vi "PDE_State_Machine_12_12_ver_3.vi"() -> ()   [LabVIEW 2016]
uses:
  PDEState.ctl
  <vilib>/DAQmx/write.llb/DAQmx Write (Digital 1D Bool NChan 1Samp 1Line).vi
  <vilib>/DAQmx/read.llb/DAQmx Read (Analog 1D Wfm NChan NSamp).vi
  StateIndicator.ctl
  SubVIs/FireSlider.ctl
panel:
  out "error out":errorcluster
  out "Temperature":waveform(dbl)[](graph)
  out "PDE Progress":dbl(slide) scale=0.0..1.0
  out "Predet Progress":dbl(slide) scale=0.0..1.0
  in  "Number of Predet Fires":T1=1 min=0 max=100 step=1 scale=1.0..100.0
  out "Predet Fire Counter":i32
  out "Pressure":waveform(dbl)[](graph)
  out "PD Values":dbl[](array[numeric])
  out "PDE State":T2 items=["Stop VI", "Predet Fire", "Control Button", "Stop", "Connecting", "Firing", "Testing ", "Idle", "Init"]
  in  "Number of Fires":T1=1 min=0 max=100 step=1 scale=1.0..100.0
  out "Fire Counter":i32
  in  "Save Data":bool
  in  "Purge":bool=TRUE
  in  "Data Time":dbl=1.0 min=0.0 max=120.0
  in  "PT Filepath":path=path "D:/PDE Project/PDE Data/Default Data/PT.tdms"
  in  "TC Filepath":path=path "D:/PDE Project/PDE Data/Default Data/TC.tdms"
  in  "PD Filepath":path=path "D:/PDE Project/PDE Data/Default Data/PD.tdms"
  in  "Valve Buttons":bool[](array[boolean])
  in  "Predet Fire Button":bool
  in  "Control Buttons":bool
  in  "PDE Fire Button":bool
  in  "Test Button":bool
  in  "Go To Idle":bool
  in  "Abort VI":bool
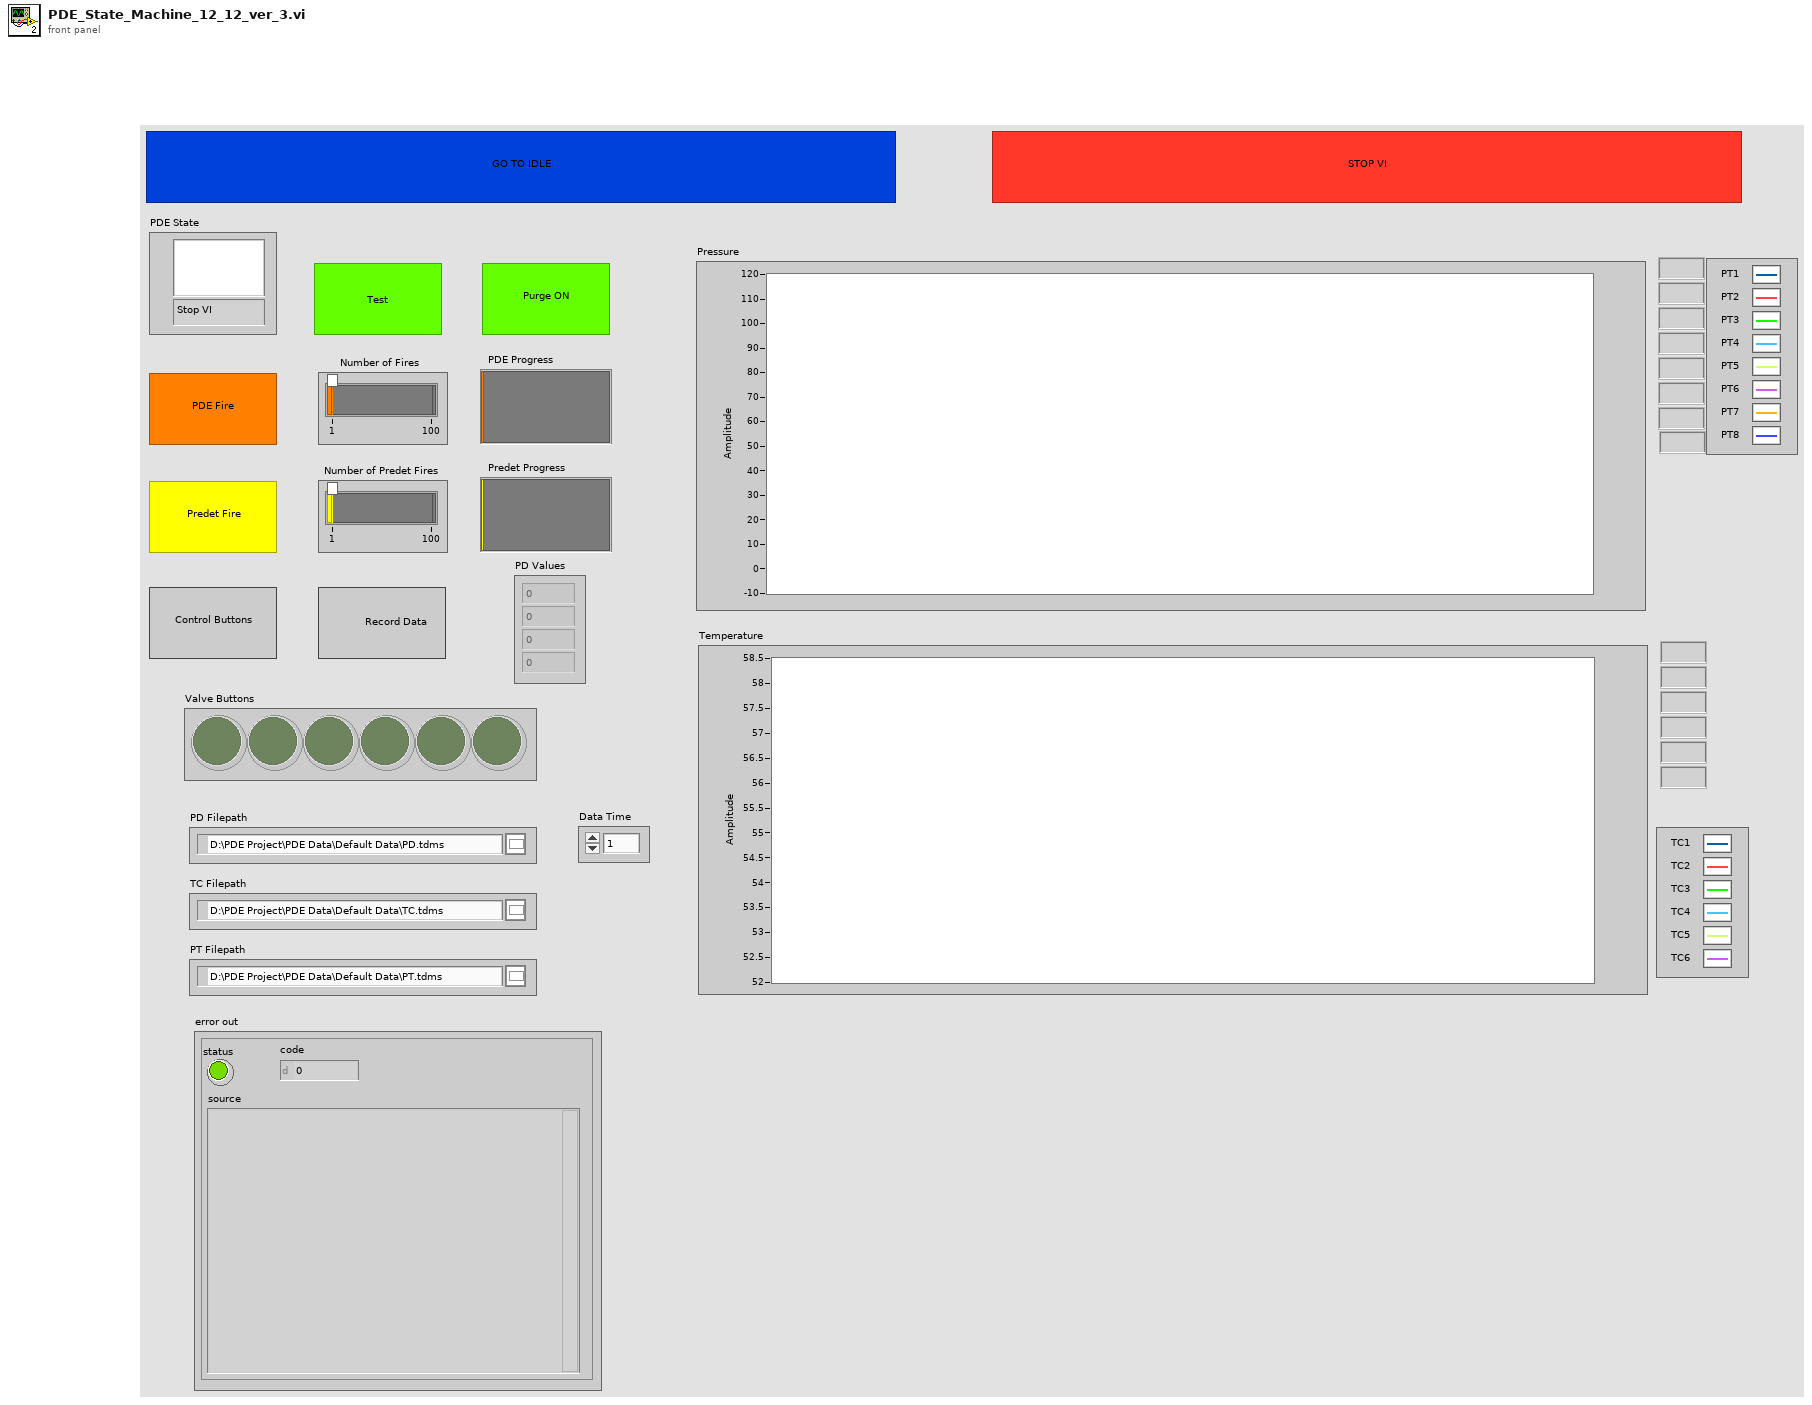
[diagram p1: front panel]
types:
  T1 = typedef "FireSlider.ctl" = i32
  T2 = typedef "StateIndicator.ctl" = u16
  T3 = typedef "PDEState.ctl" = enum16{"Stop VI", "Predet Fire", "Control Button", "Stop", "Connecting", "Firing ", "Testing ", "Idle", "Init"}
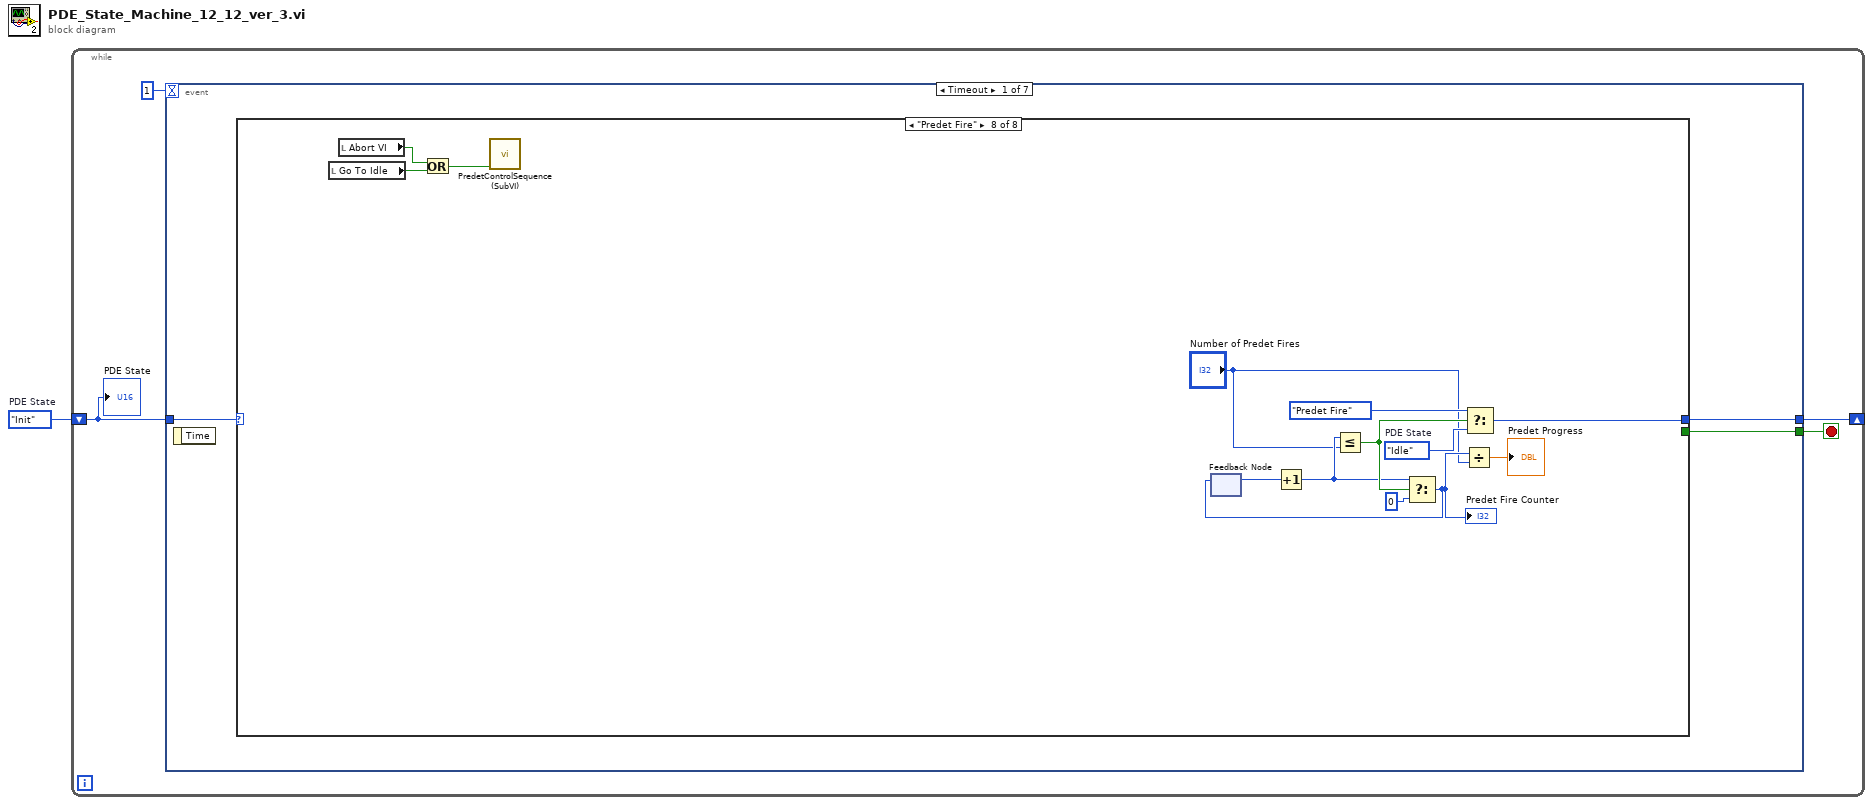
[diagram p0: block diagram]
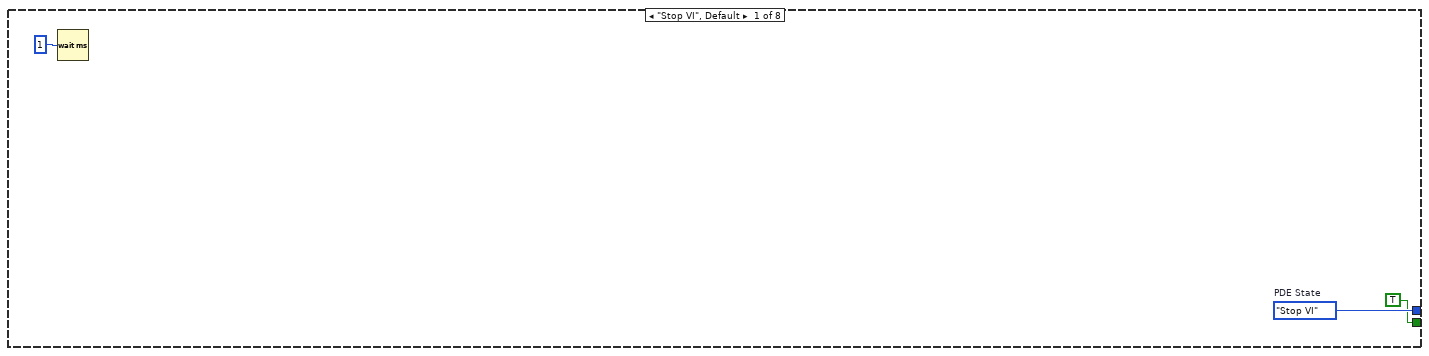
[diagram p2: hidden frame]
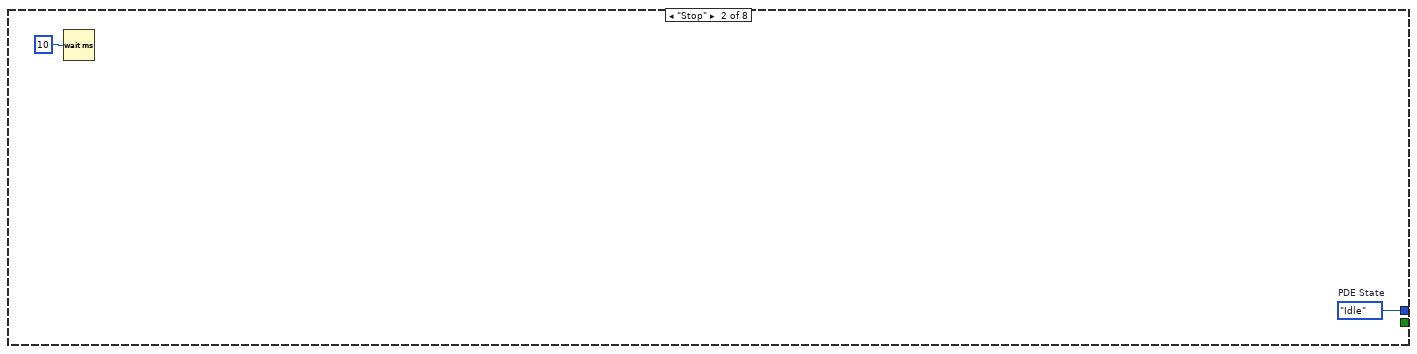
[diagram p3: hidden frame]
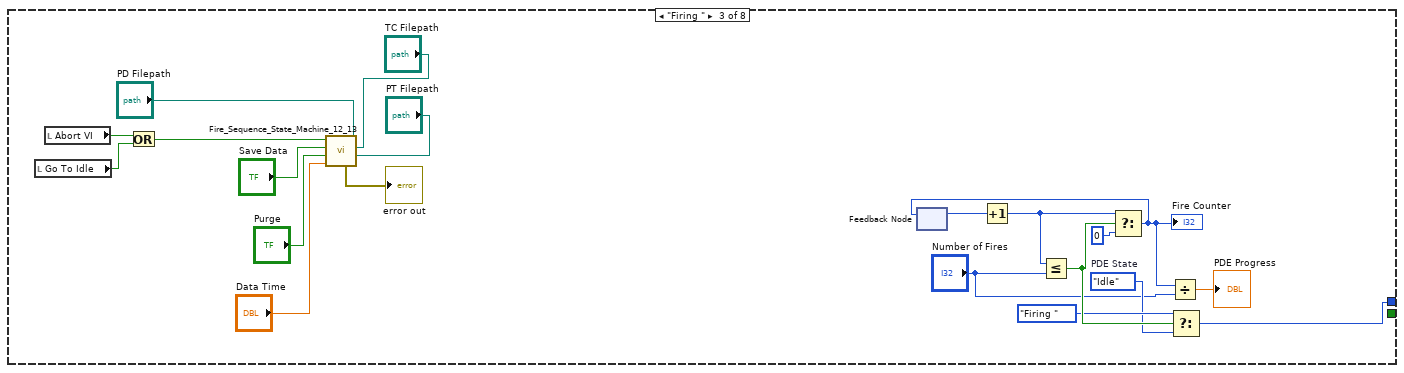
[diagram p4: hidden frame]
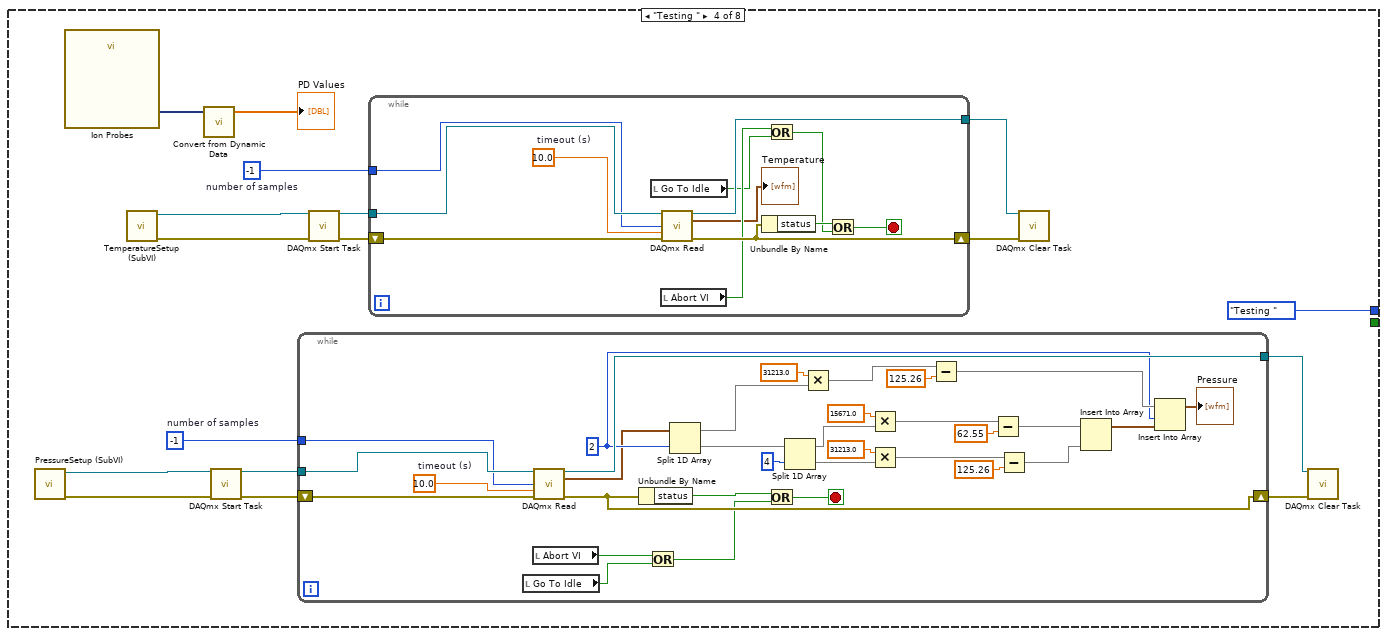
[diagram p5: hidden frame]
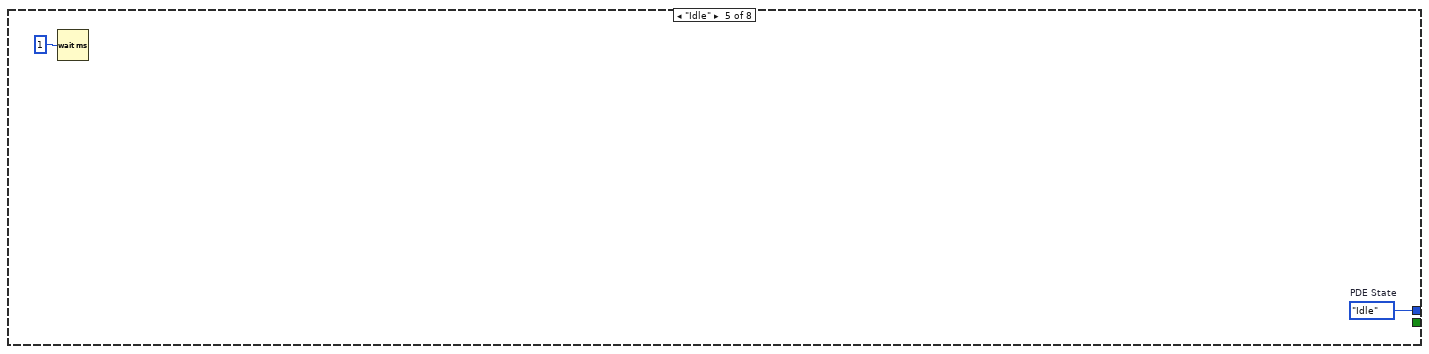
[diagram p6: hidden frame]
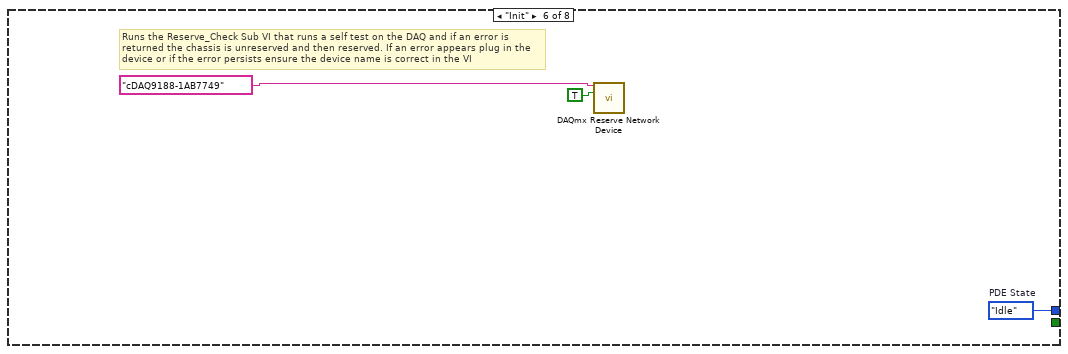
[diagram p7: hidden frame]
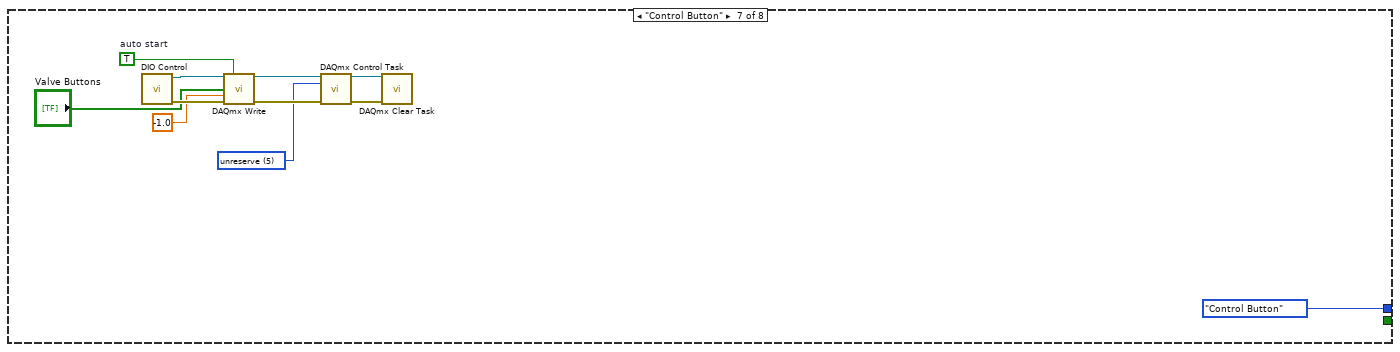
[diagram p8: hidden frame]
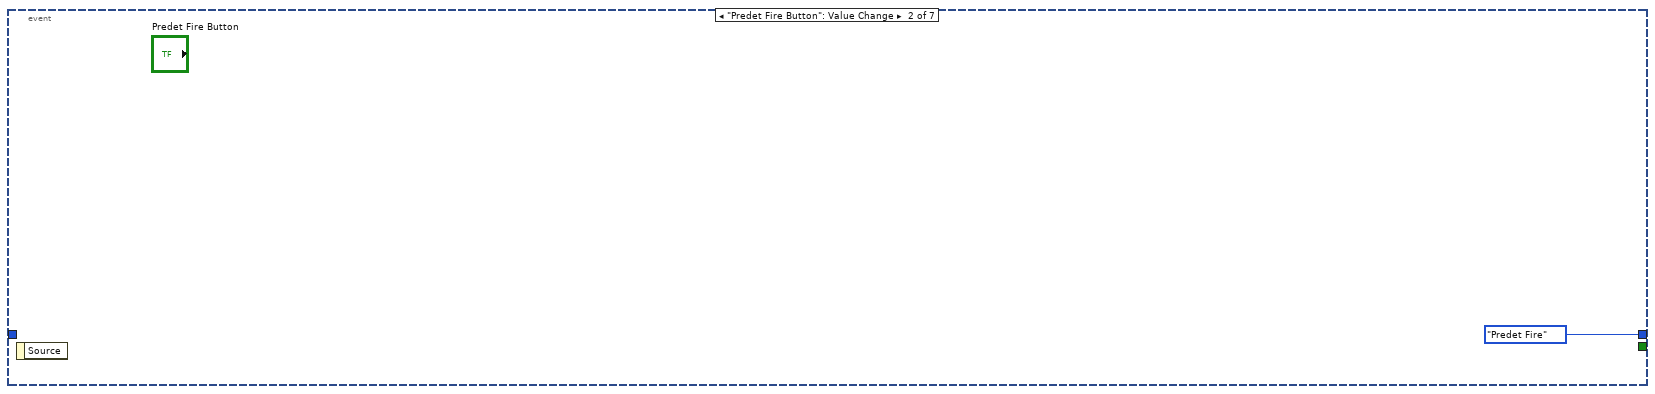
[diagram p9: hidden frame]
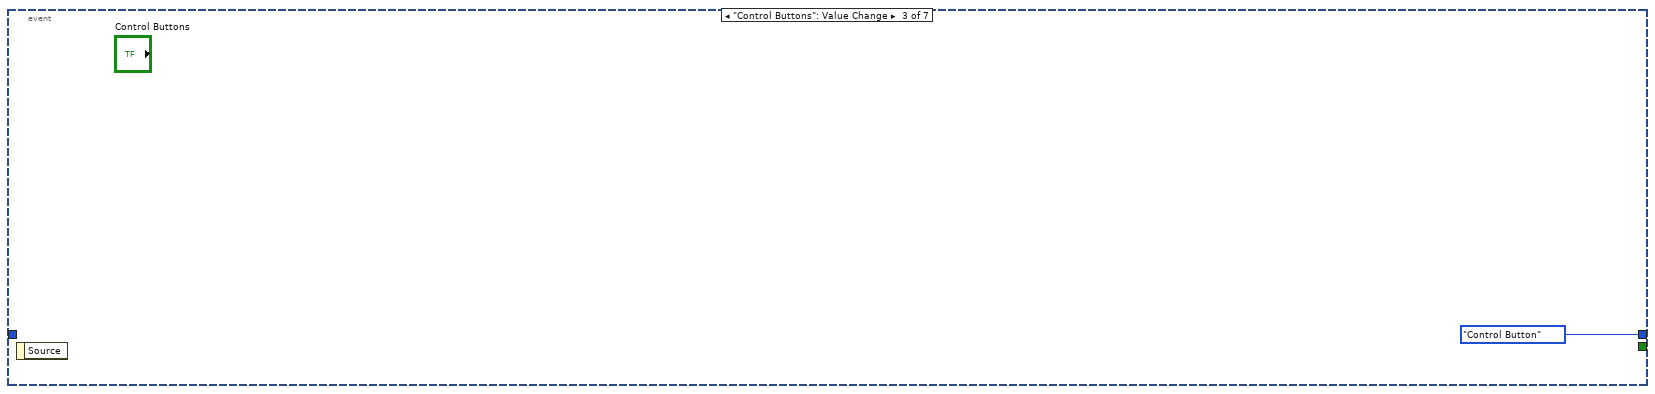
[diagram p10: hidden frame]
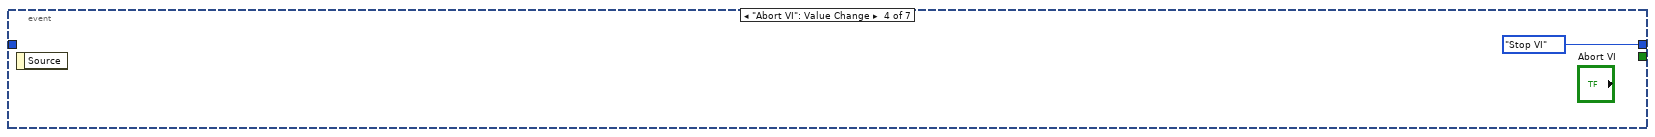
[diagram p11: hidden frame]
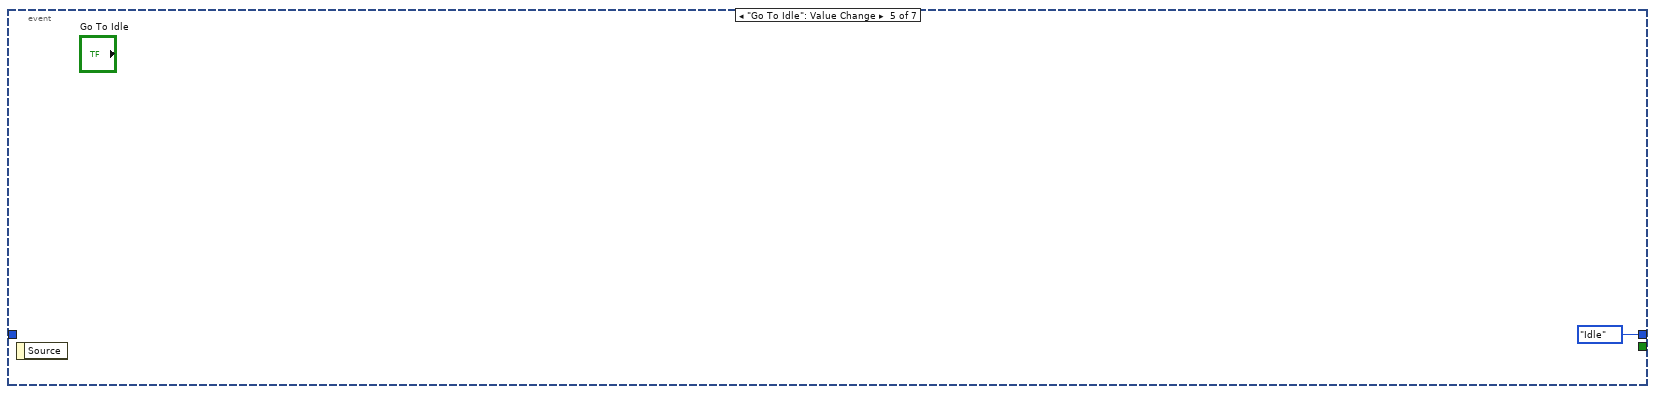
[diagram p12: hidden frame]
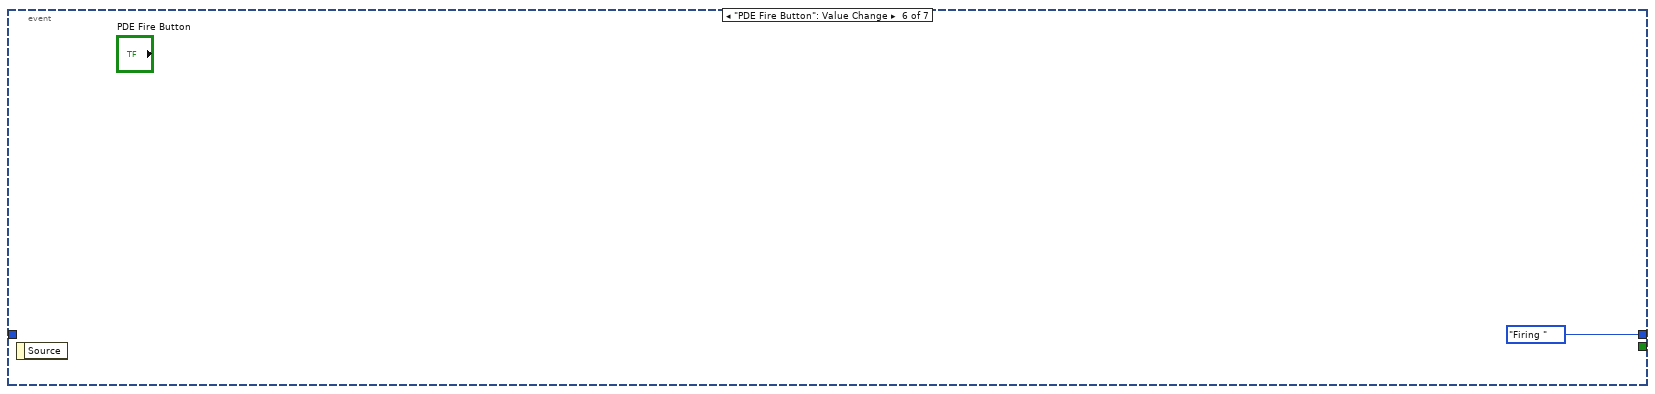
[diagram p13: hidden frame]
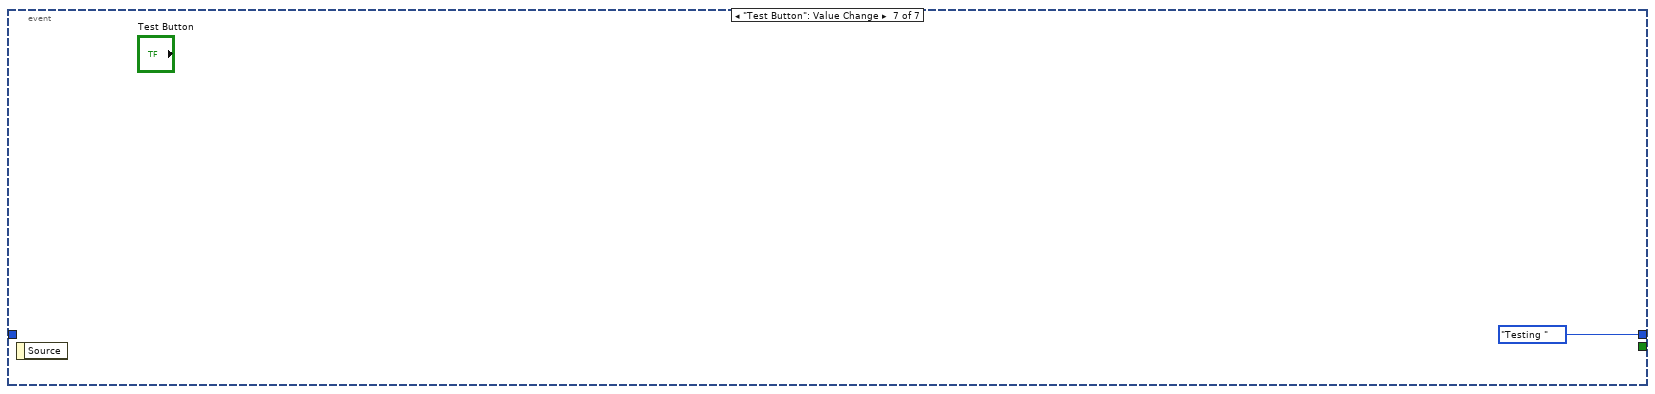
[diagram p14: hidden frame]
diagram:
  w1 = PDEState."Init"  # PDE State
  n1 = while {
    shift-right: [w4] -> _
    shift-left: w1 -> [w2]
    stop <- w3 stop-if-true
    n2 = event shown="[0] Timeout" {
      selector: _ -> [_ _ _ _ _ _ _]
      dyn-events: _ -> [_ _ _ _ _ _ _]
      timeout: 1 -> [_ _ _ _ _ _ _]
      tunnel: w2 -> [w8 _ _ _ _ _ _]
      tunnel: [w7 PDEState."Predet Fire" ("PDE State") PDEState."Control Button" ("PDE State") PDEState."Stop VI" ("PDE State") PDEState."Idle" ("PDE State") PDEState."Firing " ("PDE State") PDEState."Testing " ("PDE State")] -> w4
      tunnel: [w6 _ _ _ _ _ _] -> w3
      event Timeout {
        n3 = event-data() -> ()  [unwired: 1 in, 1 out]
        n4 = case shown="\"Predet Fire\"" w8 {
          tunnel: [w11 w13 w27 PDEState."Testing " ("PDE State") w96 w99 PDEState."Control Button" ("PDE State") w117] -> w7
          tunnel: [TRUE _ _ _ _ _ _ _] -> w6
          frame "Stop VI", Default {
            w11 = PDEState."Stop VI"  # PDE State
            n5 = Wait (ms)(milliseconds to wait=u32 1 ("millisecond timer value")) -> ()  [unwired: 1 out]
          }
          frame "Stop" {
            w13 = PDEState."Idle"  # PDE State
            n6 = Wait (ms)(milliseconds to wait=u32 10 ("millisecond timer value")) -> ()  [unwired: 1 out]
          }
          frame "Firing " {
            w28 = PDEState."Idle"  # PDE State
            n7 = local read "Go To Idle"() -> (w20:bool)
            n8 = local read "Abort VI"() -> (w19:bool)
            n9 = Or(x=w19, y=w20) -> (x .or. y?=w18:bool)
            n10 = call "Fire_Sequence_State_Machine_12_13.vi"("PT Filepath"="PT Filepath", "TC Filepath"="TC Filepath", "PD Filepath"="PD Filepath", "Data Time"="Data Time", "Purge"="Purge", "Save Data"="Save Data", "Stop Button"=w18) -> ("Error Out"=→"error out":errorcluster)  [unwired: 3 in, 1 out]
            n11 = feedback #1() -> (w31:i32)  [unwired: 1 in]
            n12 = Increment(x=w31) -> (x+1=w30:i32)
            n13 = Less Or Equal?(x=w30, y="Number of Fires") -> (x <= y?=w33:bool)
            n14 = Select(t=w30, s=w33, f=0 ("s? t:f")) -> (s? t:f=w16:i32)
            "Fire Counter" <- w16
            n15 = feedback-in #1(w16) -> ()
            n16 = Divide(x=w16, y="Number of Fires") -> (x/y=→"PDE Progress":dbl)
            n17 = Select(t=PDEState."Firing ", s=w33, f=w28) -> (s? t:f=w27:T3)
          }
          frame "Testing " {
            w38 = -1  # number of samples
            w46 = -1  # number of samples
            n18 = call "PressureSetup (SubVI).vi"() -> ("error out"=w42:errorcluster, "Refnum out"=w43:refnum<k21>)  [unwired: 10 in]
            n19 = call "Ion Probes"() -> ("data"=w49:dynamicdata)  [unwired: 17 in, 2 out]
            n20 = call "TemperatureSetup (SubVI).vi"() -> ("error out"=w34:errorcluster, "Refnum out"=w35:refnum<k21>)  [unwired: 10 in]
            n21 = call "Convert from Dynamic Data"("Dynamic Data Type"=w49) -> ("Array"=→"PD Values":dbl[])  [unwired: 3 in]
            n22 = call <vilib>:"DAQmx Start Task.vi"("task/channels in"=w43, "error in"=w42) -> ("task out"=w48:refnum<k21>, "error out"=w47:errorcluster)  [unwired: 12 out]
            n23 = while {
              tunnel: w48 -> [w94]
              tunnel: w46 -> [w91]
              tunnel: [w92] -> w44
              shift-right: [w89] -> w45
              shift-left: w47 -> [w93]
              stop <- w87 stop-if-true
              w75 = 2 ("index")
              w88 = 10.0  # timeout (s)
              n24 = local read "Go To Idle"() -> (w86:bool)
              n25 = local read "Abort VI"() -> (w85:bool)
              n26 = call-poly <vilib>:"DAQmx Read.vi"("task/channels in"=w94, "number of samples per channel"=w91, "timeout"=w88, "error in"=w93) -> ("task out"=w92:refnum<k21>, "data"=w74:waveform(dbl)[], "error out"=w89:errorcluster)  [unwired: 9 out]
              n27 = Unbundle By Name(w89) -> ("status"=w90:bool)
              n28 = Or(x=w85, y=w86) -> (x .or. y?=w84:bool)
              n29 = Split 1D Array(array=w74, index=w75) -> (first subarray=w80:waveform(dbl)[], second subarray=w72:waveform(dbl)[])
              n30 = Or(x=w90, y=w84) -> (x .or. y?=w87:bool)
              n31 = Split 1D Array(array=w72, index=4) -> (first subarray=w64:waveform(dbl)[], second subarray=w65:waveform(dbl)[])
              n32 = Multiply(x=31213.0, y=w80) -> (x*y=w83:waveform(dbl)[])
              n33 = Multiply(x=15671.0, y=w64) -> (x*y=w79:waveform(dbl)[])
              n34 = Multiply(x=31213.0, y=w65) -> (x*y=w70:waveform(dbl)[])
              n35 = Subtract(x=w83, y=125.26) -> (x-y=w76:waveform(dbl)[])
              n36 = Subtract(x=w79, y=62.55) -> (x-y=w63:waveform(dbl)[])
              n37 = Subtract(x=w70, y=125.26) -> (x-y=w66:waveform(dbl)[])
              n38 = Insert Into Array(array=w63, new element=w66) -> (w67:waveform(dbl)[])  [unwired: 1 in]
              n39 = Insert Into Array(array=w76, index=w75, new element=w67) -> (→"Pressure":waveform(dbl)[])
            }
            n40 = call <vilib>:"DAQmx Start Task.vi"("task/channels in"=w35, "error in"=w34) -> ("task out"=w40:refnum<k21>, "error out"=w39:errorcluster)  [unwired: 12 out]
            n41 = while {
              tunnel: w40 -> [w62]
              tunnel: w38 -> [w59]
              tunnel: [w60] -> w36
              shift-right: [w57] -> w37
              shift-left: w39 -> [w61]
              stop <- w56 stop-if-true
              w55 = 10.0  # timeout (s)
              n42 = local read "Go To Idle"() -> (w53:bool)
              n43 = local read "Abort VI"() -> (w54:bool)
              n44 = call-poly <vilib>:"DAQmx Read.vi"("task/channels in"=w62, "number of samples per channel"=w59, "timeout"=w55, "error in"=w61) -> ("task out"=w60:refnum<k21>, "data"=→"Temperature":waveform(dbl)[], "error out"=w57:errorcluster)  [unwired: 9 out]
              n45 = Unbundle By Name(w57) -> ("status"=w58:bool)
              n46 = Or(x=w54, y=w53) -> (x .or. y?=w52:bool)
              n47 = Or(x=w58, y=w52) -> (x .or. y?=w56:bool)
            }
            n48 = call <vilib>:"DAQmx Clear Task.vi"("task in"=w36, "error in"=w37) -> ()  [unwired: 14 out]
            n49 = call <vilib>:"DAQmx Clear Task.vi"("task in"=w44, "error in"=w45) -> ()  [unwired: 14 out]
          }
          frame "Idle" {
            w96 = PDEState."Idle"  # PDE State
            n50 = Wait (ms)(milliseconds to wait=u32 1 ("millisecond timer value")) -> ()  [unwired: 1 out]
          }
          frame "Init" {
            w99 = PDEState."Idle"  # PDE State
            # "Runs the Reserve_Check Sub VI that runs a self test on the DAQ and if an error is returned the chassis is unreserved and then reserved. If an error appears plug in the device or if the error persists ensure the device name is correct in the VI"
            n51 = call <vilib>:"DAQmx Reserve Network Device.vi"("device in"=tag "cDAQ9188-1AB7749", "override reservation?"=TRUE) -> ()  [unwired: 12 in, 2 out]
          }
          frame "Control Button" {
            w104 = 5 items=["verify"=2, "reserve"=4, "commit"=3, "unreserve"=5, "abort"=6] ("action")
            w109 = TRUE  # auto start
            n52 = call "DIO Control.vi"() -> ("error out"=w107:errorcluster, "task out"=w108:refnum<k21>)  [unwired: 10 in]
            n53 = call-poly <vilib>:"DAQmx Write.vi"("task/channels in"=w108, "auto start"=w109, "data"="Valve Buttons", "timeout"=-1.0, "error in"=w107) -> ("task out"=w106:refnum<k21>, "error out"=w105:errorcluster)  [unwired: 8 in, 1 out]
            n54 = call <vilib>:"DAQmx Control Task.vi"("task/channels in"=w106, "action"=w104, "error in"=w105) -> ("task out"=w103:refnum<k21>, "error out"=w102:errorcluster)  [unwired: 11 in]
            n55 = call <vilib>:"DAQmx Clear Task.vi"("task in"=w103, "error in"=w102) -> ()  [unwired: 13 in, 1 out]
          }
          frame "Predet Fire" {
            w118 = PDEState."Idle"  # PDE State
            n56 = local read "Go To Idle"() -> (w115:bool)
            n57 = local read "Abort VI"() -> (w116:bool)
            n58 = Or(x=w116, y=w115) -> (x .or. y?=w114:bool)
            n59 = call "PredetControlSequence (SubVI).vi"("Stop Button"=w114) -> ()  [unwired: 10 in, 1 out]
            n60 = feedback #2() -> (w121:i32)  [unwired: 1 in]
            n61 = Increment(x=w121) -> (x+1=w120:i32)
            n62 = Less Or Equal?(x=w120, y="Number of Predet Fires") -> (x <= y?=w123:bool)
            n63 = Select(t=w120, s=w123, f=0 ("s? t:f")) -> (s? t:f=w113:i32)
            "Predet Fire Counter" <- w113
            n64 = feedback-in #2(w113) -> ()
            n65 = Divide(x=w113, y="Number of Predet Fires") -> (x/y=→"Predet Progress":dbl)
            n66 = Select(t=PDEState."Predet Fire", s=w123, f=w118) -> (s? t:f=w117:T3)
          }
        }
      }
      event "Predet Fire Button": Value Change {
        n67 = event-data() -> ()  [unwired: 1 in, 1 out]
      }
      event "Control Buttons": Value Change {
        n68 = event-data() -> ()  [unwired: 1 in, 1 out]
      }
      event "Abort VI": Value Change {
        n69 = event-data() -> ()  [unwired: 1 in, 1 out]
      }
      event "Go To Idle": Value Change {
        n70 = event-data() -> ()  [unwired: 1 in, 1 out]
      }
      event "PDE Fire Button": Value Change {
        n71 = event-data() -> ()  [unwired: 1 in, 1 out]
      }
      event "Test Button": Value Change {
        n72 = event-data() -> ()  [unwired: 1 in, 1 out]
      }
    }
    "PDE State" <- w2
  }
